vi "Send Log Data.vi"(11 "signal in":waveform(dbl)) -> ()   [LabVIEW 2020, in "Acquisition whit helper loop.lvlib"]
uses:
  Acquisition whit helper loop.lvlib
  <vilib>/measure/matone.llb/Extract Single Tone Information 1 Chan.vi
  <vilib>/measure/NI_MAPro.lvlib
  Logging/Logging.lvlib
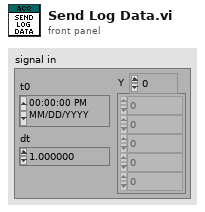
[diagram p1: front panel]
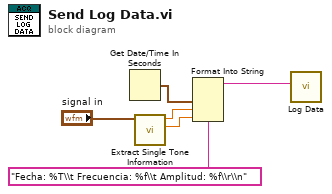
[diagram p0: block diagram]
diagram:
  n1 = Get Date/Time In Seconds() -> (seconds since 1Jan1904=w3:timestamp)
  n2 = call-poly <vilib>:"Extract Single Tone Information.vi"("time signal in"="signal in") -> ("detected amplitude"=w5:dbl, "detected frequency"=w4:dbl)  [unwired: 5 in, 4 out]
  n3 = Format Into String(format string="Fecha: %T\\t Frecuencia: %f\\t Amplitud: %f\\r\\n", w3, w4, w5) -> (resulting string=w1:string)  [unwired: 2 in, 1 out]
  n4 = call "Log Data.vi"("Data"=w1) -> ()  [unwired: 10 in, 1 out]
